vi "Get Minimal Array Properties.vi"(0 "Array Reference":refnum<vi>, 4 "Coords of Click":T1, 5 "error in":errorcluster) -> (14 "dup Array Reference":refnum<vi>, 16 "Minimal Array Properties.Bounds":T3, 17 "Minimal Array Properties.Position":T2, 18 "dup Coords of Click":T1, 19 "error out":errorcluster)   [LabVIEW 2020, in "Determine Clicked Array Element Index.lvlib"]
doc: "Determine Clicked Array Element Index - Get Minimal Array Properties.vi\n\nDescription:\nThis VI returns the minimal properties of the array specified by the Array Reference input. Minimal properties are the properties when the scrollbars, index display, label and caption are hidden.\n\nInputs:\nArray Reference - Reference to the array to operate on.\n\nCoords of Click - The coordinates indicating where the user clicked.\n\nerror in - Standard error cluster.\n\nOutputs:\ndup Array Reference - Dup reference to the array to operate on.\n\nMinimal Array Properties.Bounds - The bounds of the array when the scrollbars, index display, label and caption are hidden.\n\nMinimal Array Properties.Position - The position of the array when the scrollbars, index display, label and caption are hidden.\n\ndup Coords of Click - Dup coordinates indicating where the user clicked.\n\nerror out - Standard error cluster.\n\nDeveloped By:\nMark.ridgley\nMark.Ridgley_LabVIEW.Developer@comcast.net"
uses:
  Determine Clicked Array Element Index.lvlib
  <vilib>/Utility/miscctls.llb/LVBoundsTypeDef.ctl
  <vilib>/Utility/miscctls.llb/LVPositionTypeDef.ctl
  <vilib>/Utility/miscctls.llb/LVPoint32TypeDef.ctl
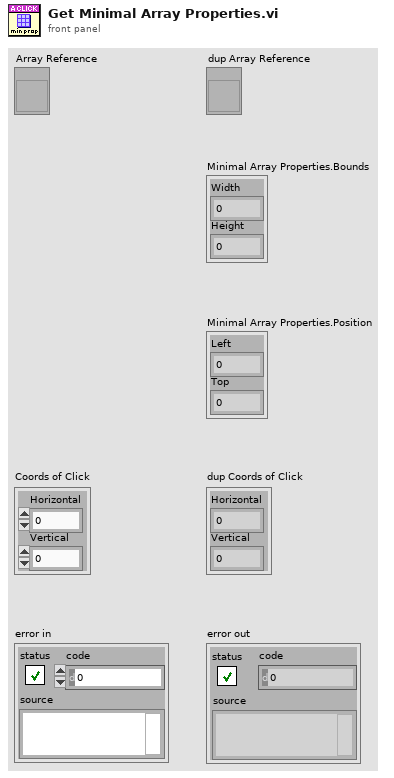
[diagram p1: front panel]
types:
  T1 = typedef "LVPoint32TypeDef.ctl" = cluster{"Horizontal":i32, "Vertical":i32}
  T2 = typedef "LVPositionTypeDef.ctl" = cluster{"Left":i32, "Top":i32}
  T3 = typedef "LVBoundsTypeDef.ctl" = cluster{"Width":u32, "Height":u32}
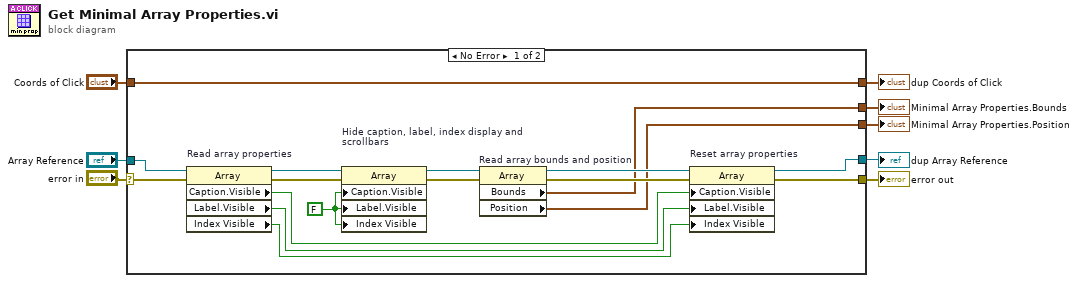
[diagram p0: block diagram]
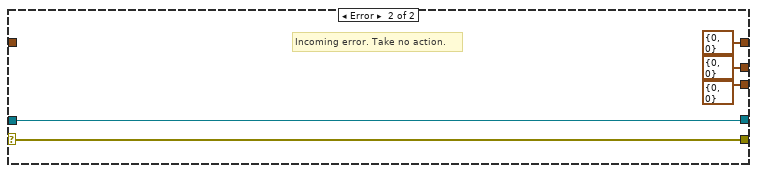
[diagram p2: hidden frame]
diagram:
  n1 = case shown="No Error" "error in" {
    selector: "error in" -> [w24 w30]
    tunnel: [w20 w29] -> w6
    tunnel: [w9 T3 {"Width"=0, "Height"=0}] -> w5
    tunnel: "Array Reference" -> [w17 w29]
    tunnel: [w13 T2 {"Left"=0, "Top"=0} ("Position")] -> w3
    tunnel: [w23 w30] -> w7
    tunnel: [w12 T1 {"Horizontal"=0, "Vertical"=0} ("Coords of Click")] -> w2
    tunnel: "Coords of Click" -> [w12 _]
    frame No Error {
      w10 = FALSE ("Label.Visible")
      n2 = property on="Read array properties" class="Array"(reference=w17, error in=w24) -> (reference out=w11:refnum<vi>, error out=w21:errorcluster, "Caption.Visible"=w14:bool, "Label.Visible"=w15:bool, "Index Visible"=w19:bool)
      n3 = property on="Hide caption, label, index display and scrollbars" class="Array"(reference=w11, error in=w21, "Caption.Visible"=w10, "Label.Visible"=w10, "Index Visible"=w10) -> (reference out=w18:refnum<vi>, error out=w22:errorcluster)
      n4 = property on="Read array bounds and position" class="Array"(reference=w18, error in=w22) -> (reference out=w16:refnum<vi>, error out=w25:errorcluster, "Bounds"=w9:T3, "Position"=w13:T2)
      n5 = property on="Reset array properties" class="Array"(reference=w16, error in=w25, "Caption.Visible"=w14, "Label.Visible"=w15, "Index Visible"=w19) -> (reference out=w20:refnum<vi>, error out=w23:errorcluster)
    }
    frame Error {
      # "Incoming error. Take no action."
    }
  }
  "dup Array Reference" <- w6
  "Minimal Array Properties.Bounds" <- w5
  "Minimal Array Properties.Position" <- w3
  "error out" <- w7
  "dup Coords of Click" <- w2
